vi "Group_FromClass.vi"(8 "error in (no error)":errorcluster, 10 "Group.lvclass":refnum<class "Group.lvclass">, 11 "Node Ptr":T1 format="%.0x") -> (0 "error out":errorcluster, 2 "Group Ref":T1=18446744073709551615 format="%.0x", 3 "Node Ptr Out":T1 format="%.0x")   [LabVIEW 2024, in "Embedded TDMS Logger System Explorer.lvlib"]
doc: "Creates a group section in the VeriStand System Definition File Custom Device based on a Group definition of the Group and subsequently creates the channels based on the channel classes stored as children within the group class."
uses:
  Embedded TDMS Logger System Explorer.lvlib
  <vilib>/NI VeriStand/Custom Device API/Custom Device Item Ref.ctl
  Shared/File Classes/Group/Group.lvclass
  Shared/Constants.vi
  <vilib>/NI VeriStand/Custom Device API/Set Item Property (Variant).vi
  <vilib>/NI VeriStand/Custom Device API/Custom Device API.lvlib
  Shared/Embedded TDMS Logger Shared.lvlib
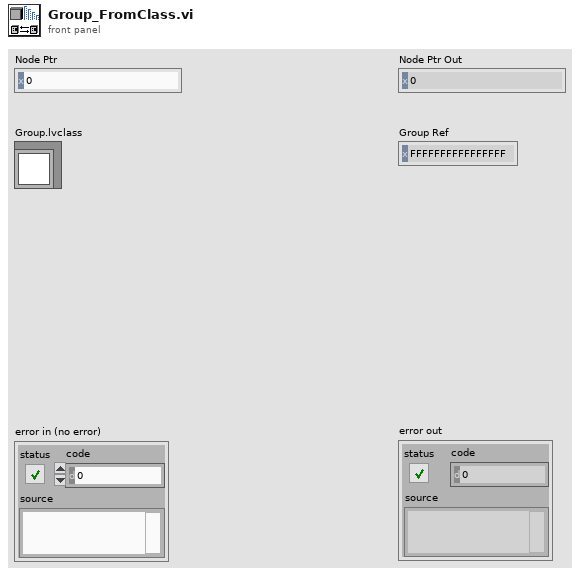
[diagram p1: front panel]
types:
  T1 = typedef "Custom Device API.lvlib/Custom Device Item Ref.ctl" = u64
  T2 = typedef "Meta Data.ctl" = cluster{"Key":string, "Value":string}
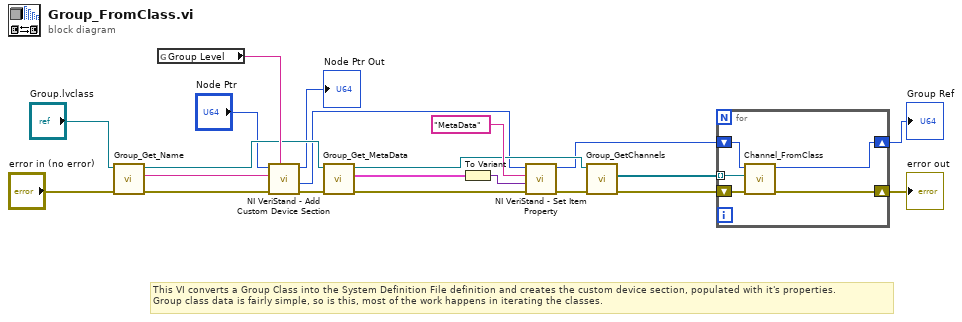
[diagram p0: block diagram]
diagram:
  # "This VI converts a Group Class into the System Definition File definition and creates the custom device section, populated with it's properties.\nGroup class data is fairly simple, so is this, most of the work happens in iterating the classes."
  n1 = call-dynamic "Group_Get_Name.vi"("error in (no error)"="error in (no error)", "Group in"="Group.lvclass") -> ("error out"=w18:errorcluster, "Name"=w20:string, "Group out"=w13:refnum<class "Group.lvclass">)  [unwired: 7 in]
  n2 = global read "Constants.vi" "Group Level"() -> (w19:string)
  n3 = call <vilib>:"NI VeriStand - Add Custom Device Section.vi"("GUID (Default Section)"=w19, "error in (no error)"=w18, "Section Name"=w20, "Parent Ref in"="Node Ptr") -> ("error out"=w12:errorcluster, "Section Ptr"=w3:T1, "Parent Ref out"=→"Node Ptr Out":T1)  [unwired: 4 in, 1 out]
  n4 = call-dynamic "Group_Get_MetaData.vi"("error in (no error)"=w12, "Group in"=w13) -> ("error out"=w14:errorcluster, "Meta Data"=w15:T2[], "Group out"=w8:refnum<class "Group.lvclass">)  [unwired: 7 in]
  n5 = To Variant(anything=w15) -> (Variant=w6:variant)
  n6 = call-poly <vilib>:"NI VeriStand - Set Item Property.vi"("error in (no error)"=w14, "Value"=w6, "Property Name"="MetaData", "Item Ref in"=w3) -> ("error out"=w10:errorcluster, "Item Ref out"=w1:T1)  [unwired: 5 in, 1 out]
  n7 = call-dynamic "Group_GetChannels.vi"("error in (no error)"=w10, "Group in"=w8) -> ("error out"=w9:errorcluster, "Channels"=w11:refnum<class "Channel.lvclass">[])  [unwired: 7 in, 1 out]
  n8 = for {
    tunnel: w11 -> [w26] mode=indexing
    shift-right: [w23] -> w7
    shift-left: w9 -> [w24]
    shift-right: [w22] -> w4
    shift-left: w1 -> [w25]
    n9 = call "Channel_FromClass.vi"("error in (no error)"=w24, "Channel.lvclass"=w26, "Node Ptr"=w25) -> ("error out"=w23:errorcluster, "Node Ptr Out"=w22:T1)  [unwired: 6 in, 1 out]
  }
  "error out" <- w7
  "Group Ref" <- w4
